vi "MD5-Hashing.vi"() -> ()   [LabVIEW 2019]
uses:
  07ca0bf1-60f3-4af8-95f0-d570cf04a382.vi
panel:
  in  "text":string
  out "MD5 message-digest":string
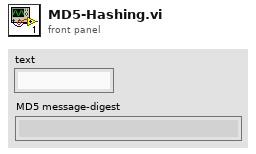
[diagram p1: front panel]
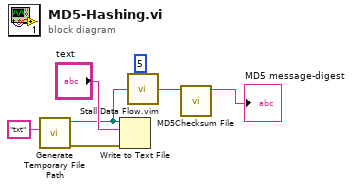
[diagram p0: block diagram]
diagram:
  n1 = call <vilib>:"Generate Temporary File Path.vi"("Temporary File Extension (tmp)"="txt") -> ("error out"=w5:errorcluster, "Unique Temporary File Path"=w2:path)  [unwired: 9 in]
  n2 = Write to Text File(file (use dialog)=w2, text="text", error in=w5) -> ()  [unwired: 1 in, 3 out]
  n3 = call "Stall Data Flow.vim"("value in"=w2, "milliseconds to wait"=u32 5) -> ("value out"=w3:path)  [unwired: 1 out]
  n4 = call <vilib>:"MD5Checksum File.vi"("Path"=w3) -> ("MD5 message-digest"=→"MD5 message-digest":string)  [unwired: 9 in, 1 out]
